vi "SVFA Magnitude and Phase to Real and Imaginary (1 Ch).vi"(0 "magnitude spectrum":cluster{"x0":dbl, "dx":dbl, "magnitude":dbl[]}, 2 "phase spectrum":cluster{"x0":dbl, "dx":dbl, "phase":dbl[]}, 4 "spectrum info in":T1={"channel name"="", "description"="", "x-axis units"=0, "spectral info"={"spectrum type"=enum."Power [Magnitude^2]", "linear/dB"=enum."linear", "window"=0, "window size"=0, "FFT size"=0}, "engineering units"=0, "custom label"="", "dB reference [EU]"=0.0, "peak units"=enum."rms", "weighting filter"=0, "spectral density?"=FALSE, "unit label"="", "spectrum skewed?"=FALSE, "complimentary spectrum units"=enum."none"} {"x-axis units" items=["Time (s)"=0, "Frequency-CB (Hz)"=1, "Frequency-CPB (Hz)"=1248, "Frequency-Arbitrary (Hz)"=2357, "Quefrency (s)"=2, "Revolutions (rev)"=3, "Order"=4, "Speed (RPM)"=11, "Speed (rad/s)"=21, "Index"=65535]; "weighting filter" items=["Linear", "A-weighting", "B-weighting", "C-weighting", "ITU-R 468-4", "Dolby", "CCITT", "C-message", "Wb", "Wc", "Wd", "We", "Wf", "Wh", "Wj", "Wk", "Wm", "AES17 20 kHz lowpass", "AES17 40 kHz lowpass", "AES17 20 kHz highpass", "AES17 40 kHz highpass"]; "dB reference [EU]" format="%.2f"; "engineering units" items=["custom..."=0, "V"=1, "A"=21, "C"=30, "pC"=31, "s"=32, "-"=29, "Pa"=2, "N"=20, "g"=3, "m/s^2"=4, "m/s"=5, "m"=6, "mm/s"=12, "mm"=13, "micron/s"=14, "micron"=15, "in/s^2"=7, "in/s"=8, "in"=9, "mil/s"=10, "mil"=11, "rad/s^2"=16, "rad/s"=17, "rad"=18, "deg/s^2"=26, "deg/s"=27, "deg"=28, "RPM"=22, "cycle/s^2"=23, "Hz"=24, "cycle"=25, "strain"=19]; "spectral info"."window" items=["None "=0, "Hanning"=1, "Hamming"=2, "Blackman-Harris"=3, "Exact Blackman"=4, "Blackman"=5, "Flat Top"=6, "4 Term B-Harris "=7, "7 Term B-Harris"=8, "Low Sidelobe"=9, "Force - Exponential"=10, "Gaussian"=62]}, 5 "error in (no error)":errorcluster) -> (12 "Nyquist plot":T8, 14 "real spectrum":cluster{"x0":dbl, "dx":dbl, "real part":dbl[]}, 16 "imaginary spectrum":T7, 17 "unit label":string, 18 "spectrum info out":T1={"channel name"="", "description"="", "x-axis units"=0, "spectral info"={"spectrum type"=enum."Power [Magnitude^2]", "linear/dB"=enum."linear", "window"=0, "window size"=0, "FFT size"=0}, "engineering units"=1, "custom label"="", "dB reference [EU]"=0.0, "peak units"=enum."rms", "weighting filter"=0, "spectral density?"=FALSE, "unit label"="", "spectrum skewed?"=FALSE, "complimentary spectrum units"=enum."none"} {"x-axis units" items=["Time (s)"=0, "Frequency-CB (Hz)"=1, "Frequency-CPB (Hz)"=1248, "Frequency-Arbitrary (Hz)"=2357, "Quefrency (s)"=2, "Revolutions (rev)"=3, "Order"=4, "Speed (RPM)"=11, "Speed (rad/s)"=21, "Index"=65535]; "weighting filter" items=["Linear", "A-weighting", "B-weighting", "C-weighting", "ITU-R 468-4", "Dolby", "CCITT", "C-message", "Wb", "Wc", "Wd", "We", "Wf", "Wh", "Wj", "Wk", "Wm", "AES17 20 kHz lowpass", "AES17 40 kHz lowpass", "AES17 20 kHz highpass", "AES17 40 kHz highpass"]; "dB reference [EU]" format="%.2f"; "engineering units" items=["custom..."=0, "V"=1, "A"=21, "C"=30, "pC"=31, "s"=32, "-"=29, "Pa"=2, "N"=20, "g"=3, "m/s^2"=4, "m/s"=5, "m"=6, "mm/s"=12, "mm"=13, "micron/s"=14, "micron"=15, "in/s^2"=7, "in/s"=8, "in"=9, "mil/s"=10, "mil"=11, "rad/s^2"=16, "rad/s"=17, "rad"=18, "deg/s^2"=26, "deg/s"=27, "deg"=28, "RPM"=22, "cycle/s^2"=23, "Hz"=24, "cycle"=25, "strain"=19]; "spectral info"."window" items=["None "=0, "Hanning"=1, "Hamming"=2, "Blackman-Harris"=3, "Exact Blackman"=4, "Blackman"=5, "Flat Top"=6, "4 Term B-Harris "=7, "7 Term B-Harris"=8, "Low Sidelobe"=9, "Force - Exponential"=10, "Gaussian"=62]}, 19 "error out":errorcluster)   [LabVIEW 2017]
doc: "Converts spectra from polar components to rectangular components. This conversion can reduce the computational power necessary to view and process spectra. Wire data to the <B>magnitude spectrum</B> and <B>phase spectrum</B> inputs to determine the polymorphic instance to use or manually select the instance."
uses:
  <vilib>/addons/_NISVFA/_Shared subVIs/Controls/svc_Spectrum Info.ctl
  <vilib>/addons/_NISVFA/_Shared subVIs/Controls/svc_X-Axis Units.ctl
  <vilib>/addons/_NISVFA/_Shared subVIs/Controls/svc_Spectrum Type.ctl
  <vilib>/addons/_NISVFA/_Shared subVIs/Controls/svc_Engineering Units Text Ring.ctl
  <vilib>/addons/_NISVFA/_Shared subVIs/Controls/svc_Weighting Filter Text Ring.ctl
  <vilib>/addons/_NISVFA/_Shared subVIs/Controls/svc_Complimentary Spectrum Units.ctl
  <vilib>/addons/_NISVFA/_Shared subVIs/Common/svc_Get Weighting Enum and Labels.vi
  <vilib>/addons/_NISVFA/_Shared subVIs/Common/svc_Unit Label Lexical Class.vi
  <vilib>/addons/_NISVFA/_Shared subVIs/Common/svc_Engineering Units to Unit Label.vi
  <vilib>/addons/_NISVFA/_Shared subVIs/Common/svc_Format Value (DBL).vi
  <vilib>/addons/_NISVFA/_Spectrum Processing/SVFA Phase Unit Conversion (1 Ch).vi
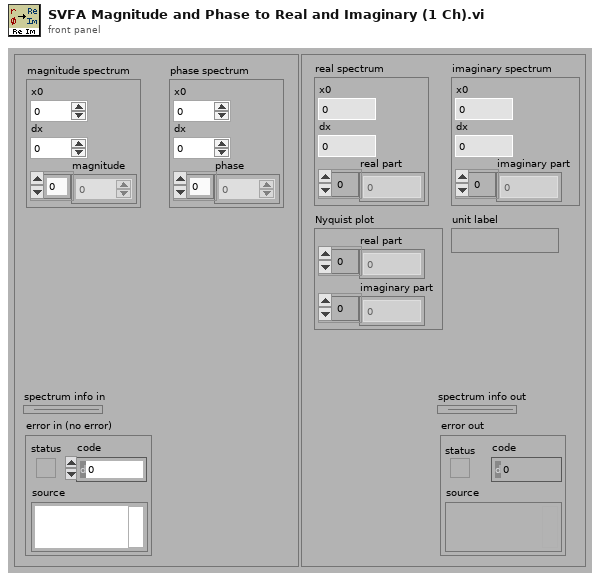
[diagram p1: front panel]
types:
  T1 = typedef "svc_Spectrum Info.ctl" = cluster{"channel name":string, "description":string, "x-axis units":T2, "spectral info":cluster{"spectrum type":T3, "linear/dB":enum16{"linear", "dB"}, "window":u16, "window size":i32, "FFT size":i32}, "engineering units":T4, "custom label":string, "dB reference [EU]":dbl, "peak units":enum16{"rms", "peak", "peak-peak"}, "weighting filter":T5, "spectral density?":bool, "unit label":string, "spectrum skewed?":bool, "complimentary spectrum units":T6}
  T2 = typedef "svc_X-Axis Units.ctl" = u16
  T3 = typedef "svc_Spectrum Type.ctl" = enum16{"FFT Spectrum [complex]", "Amplitude [Magnitude]", "Power [Magnitude^2]", "Cross Spectrum [complex]", "Frequency Response [Complex]"}
  T4 = typedef "svc_Engineering Units Text Ring.ctl" = u16
  T5 = typedef "svc_Weighting Filter Text Ring.ctl" = u16
  T6 = typedef "svc_Complimentary Spectrum Units.ctl" = enum16{"none", "radians", "degrees", "cycles", "imaginary"}
  T7 = cluster{"x0":dbl, "dx":dbl, "imaginary part":dbl[]}
  T8 = cluster{"real part":dbl[], "imaginary part":dbl[]}
  T9 = enum16{"No change", "Radians", "Degrees", "Cycles"}
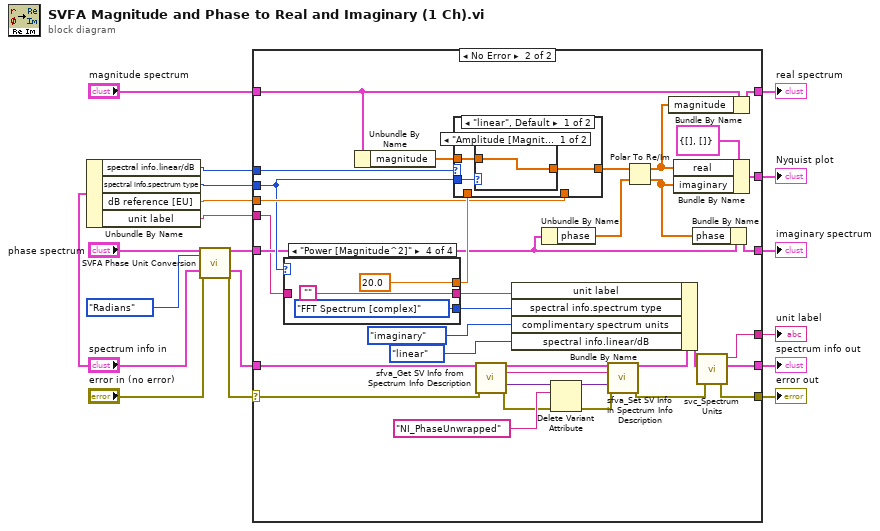
[diagram p0: block diagram]
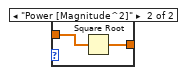
[diagram p3: hidden frame]
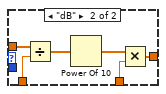
[diagram p4: hidden frame]
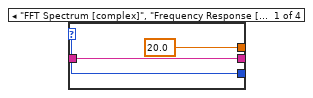
[diagram p5: hidden frame]
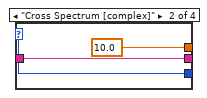
[diagram p6: hidden frame]
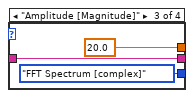
[diagram p7: hidden frame]
diagram:
  n1 = Unbundle By Name("spectrum info in") -> ("spectral info.linear/dB"=w11:enum16{"linear", "dB"}, "spectral info.spectrum type"=w12:T3, "dB reference [EU]"=w3:dbl, "unit label"=w2:string)
  n2 = call-poly <vilib>:"SVFA Phase Unit Conversion.vi"("phase spectrum"="phase spectrum", "desired units"=T9."Radians", "spectrum info in"="spectrum info in", "error in (no error)"="error in (no error)") -> ("converted phase spectrum"=w5:cluster{"f0":dbl, "df":dbl, "phase":dbl[]}, "spectrum info out"=w8:T1, "error out"=w6:errorcluster)  [unwired: 12 in, 1 out]
  n3 = case shown="No Error" w6 {
    selector: w6 -> [w19 w26]
    tunnel: [_ w55] -> w18
    tunnel: "magnitude spectrum" -> [_ w46]
    tunnel: w5 -> [_ w39]
    tunnel: [_ w54] -> w16
    tunnel: [w19 w34] -> w15
    tunnel: [_ w49] -> w14
    tunnel: [w20 w35] -> w13
    tunnel: w8 -> [w20 w28]
    tunnel: w12 -> [_ w40]
    tunnel: w3 -> [_ w43]
    tunnel: w11 -> [_ w41]
    tunnel: w2 -> [_ w38]
    tunnel: [_ w33] -> w1
    frame Error {
    }
    frame No Error {
      n4 = case shown="\"Power [Magnitude^2]\"" w40 {
        selector: w40 -> [w70 w73 _ _]
        tunnel: [w70 w73 svc_Spectrum_Type."FFT Spectrum [complex]" ("spectrum type") svc_Spectrum_Type."FFT Spectrum [complex]" ("spectrum type")] -> w48
        tunnel: [20.0 ("y") 10.0 ("y") 20.0 ("y") 20.0 ("y")] -> w44
        tunnel: [w68 w71 w74 "" ("unit label")] -> w37
        tunnel: w38 -> [w68 w71 w74 _]
        frame "FFT Spectrum [complex]", "Frequency Response [Complex]", Default {
        }
        frame "Cross Spectrum [complex]" {
        }
        frame "Amplitude [Magnitude]" {
        }
        frame "Power [Magnitude^2]" {
        }
      }
      n5 = Unbundle By Name(w46) -> ("magnitude"=w45:dbl[])
      n6 = case shown="\"linear\", Default" w41 {
        tunnel: w45 -> [w57 w67]
        tunnel: w44 -> [_ w66]
        tunnel: w43 -> [_ w63]
        tunnel: [w56 w62] -> w42
        tunnel: w40 -> [w58 _]
        frame "linear", Default {
          n7 = case shown="\"Amplitude [Magnitude]\", Default" w58 {
            tunnel: w57 -> [w59 w61]
            tunnel: [w59 w60] -> w56
            frame "Amplitude [Magnitude]", Default {
            }
            frame "Power [Magnitude^2]" {
              n8 = Square Root(x=w61) -> (sqrt(x)=w60:dbl[])
            }
          }
        }
        frame "dB" {
          n9 = Divide(x=w67, y=w66) -> (x/y=w65:dbl[])
          n10 = Power Of 10(x=w65) -> (10^x=w64:dbl[])
          n11 = Multiply(x=w64, y=w63) -> (x*y=w62:dbl[])
        }
      }
      n12 = call <vilib>:"sfva_Get SV Info from Spectrum Info Description.vi"("spectrum info"=w28, "error in (no error)"=w26) -> ("spectrum info"=w30:T1, "description"=w29:string, "SV Info"=w23:variant, "error out"=w21:errorcluster)  [unwired: 9 in, 1 out]
      n13 = Unbundle By Name(w39) -> ("phase"=w51:dbl[])
      n14 = Delete Variant Attribute(4:w21, 6:"NI_PhaseUnwrapped" ("name"), 7:w23) -> (0:w22:errorcluster, 3:w31:variant)  [unwired: 1 out]
      n15 = call <vilib>:"sfva_Set SV Info in Spectrum Info Description.vi"("spectrum info"=w30, "description"=w29, "SV Info"=w31, "error in (no error)"=w22) -> ("spectrum info"=w27:T1, "error out"=w25:errorcluster)  [unwired: 10 in]
      n16 = Bundle By Name(cluster=w27, "unit label"=w37, "spectral info.spectrum type"=w48, "complimentary spectrum units"=svc_Complimentary_Spectrum_Units."imaginary", "spectral info.linear/dB"=enum16{"linear", "dB"}."linear") -> (w36:T1)
      n17 = Polar To Re/Im(2:w51, 3:w42) -> (0:w50:dbl[], 1:w52:dbl[])
      n18 = Bundle By Name(cluster=w46, "magnitude"=w52) -> (w54:cluster{"x0":dbl, "dx":dbl, "magnitude":dbl[]})
      n19 = Bundle By Name(cluster=cluster{"real":dbl[], "imaginary":dbl[]} {"real"=[], "imaginary"=[]} ("Nyquist plot"), "real"=w52, "imaginary"=w50) -> (w55:cluster{"real":dbl[], "imaginary":dbl[]})
      n20 = Bundle By Name(cluster=w39, "phase"=w50) -> (w49:cluster{"f0":dbl, "df":dbl, "phase":dbl[]})
      n21 = call <vilib>:"svc_Spectrum Units.vi"("error in (no error)"=w25, "spectrum info in"=w36) -> ("error out"=w34:errorcluster, "spectrum info out"=w35:T1, "unit label"=w33:string)  [unwired: 2 in, 1 out]
    }
  }
  "Nyquist plot" <- w18
  "real spectrum" <- w16
  "imaginary spectrum" <- w14
  "error out" <- w15
  "spectrum info out" <- w13
  "unit label" <- w1
